vi "Write Sigle Dword.vi"(8 "error in (no error)":errorcluster, 10 "Data":u32, 11 "Tags":string) -> (0 "error out":errorcluster, 2 "Boolean":bool, 3 "Siemens Ctr out":T1)   [LabVIEW 2014]
uses:
  Simatic S7.lvlib
panel:
  in  "file path (dialog if empty)":path caption="文件路径 （空时为对话框）"
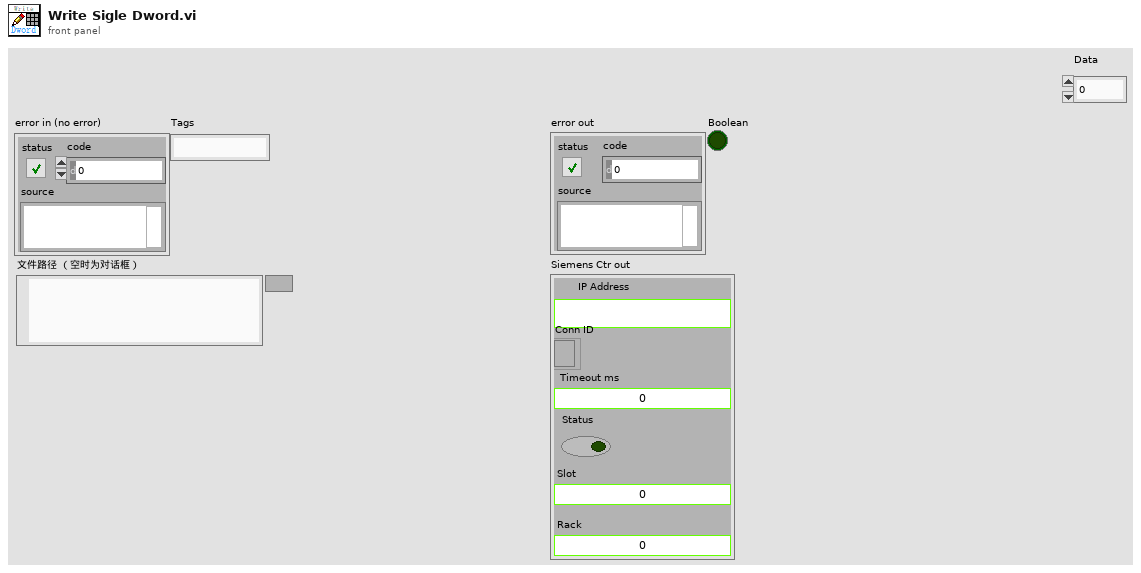
[diagram p1: front panel]
types:
  T1 = typedef "Simatic S7.lvlib/Siemens Ref.ctl" = cluster{"IP Address ":string, "Conn ID":refnum<k5>, "Timeout ms":i32, "Status":bool, "Slot":u16, "Rack":u16}
  T2 = typedef "Simatic S7.lvlib/Operation Siemens Ref.ctl" = enum16{"Init", "Add Ref", "Get Ref", "Set Error", "Close Close"}
  T3 = typedef "PLC Address.ctl" = cluster{"Address Areas":u8, "Data Type":enum8{"Bit", "Byte", "int", "Word", "Dint", "Dword", "Real", "String"}, "DB.No":u16, "Byte":u32, "Length":u16, "Item":u16}
  T4 = typedef "Semaphore RefNum" = refnum<k1>
  T5 = typedef "Simatic S7.lvlib/Op ip address.ctl" = enum16{"Init", "Add IP", "Get IP"}
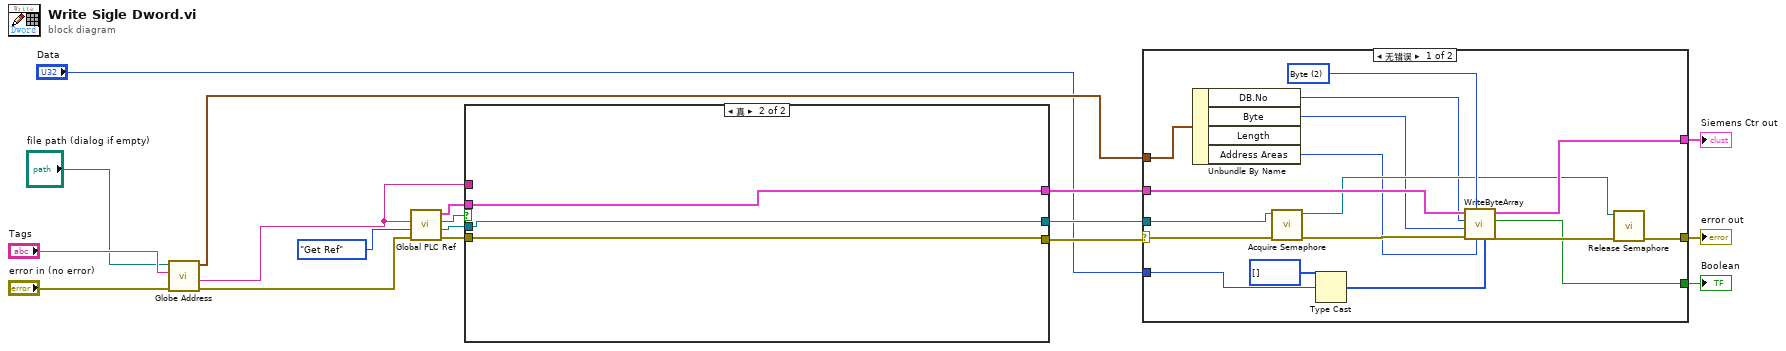
[diagram p0: block diagram]
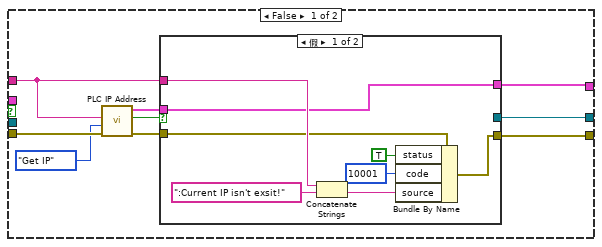
[diagram p3: hidden frame]
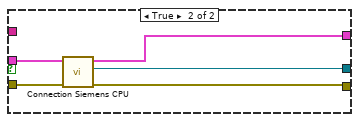
[diagram p4: hidden frame]
diagram:
  n1 = call "Globe Address.vi"("error in (no error)"="error in (no error)", "Tag"="Tags", "file path (dialog if empty)"="file path (dialog if empty)") -> ("error out"=w9:errorcluster, "IP"=w8:string, "ddress"=w6:T3)  [unwired: 5 in, 1 out]
  n2 = call "Global PLC Ref.vi"("error in (no error)"=w9, "Operation Siemens Ref"=Operation_Siemens_Ref."Get Ref", "IP Address"=w8) -> ("error out"=w16:errorcluster, "semaphore"=w14:T4, "Boolean"=w17:bool, "Siemens Ctr out"=w15:T1)  [unwired: 4 in, 1 out]
  n3 = case shown="真" w17 {
    tunnel: w16 -> [w27 w43]
    tunnel: w8 -> [w23 _]
    tunnel: [w21 w43] -> w13
    tunnel: [w20 w41] -> w12
    tunnel: [w19 w42] -> w11
    tunnel: w15 -> [_ w42]
    tunnel: w14 -> [_ w41]
    frame False {
      n4 = call "PLC IP Address.vi"("error in (no error)"=w27, "Operationip"=Op_ip_address."Get IP", "IP Address"=w23) -> ("error out"=w24:errorcluster, "Boolean"=w25:bool, "Siemens Ctr out"=w22:T1)  [unwired: 6 in]
      n5 = case shown="假" w25 {
        tunnel: w24 -> [w33 w40]
        tunnel: w23 -> [w34 _]
        tunnel: w22 -> [w28 w39]
        tunnel: [w29 w38] -> w21
        tunnel: [_ w37] -> w20
        tunnel: [w28 w36] -> w19
        frame False {
          n6 = Concatenate Strings(w34, ":Current IP isn't exsit!") -> (w31:string)
          n7 = Bundle By Name(cluster=w33, "status"=TRUE, "code"=10001, "source"=w31) -> (w29:errorcluster)
        }
        frame True {
          n8 = call "Connection Siemens CPU.vi"("error in (no error)"=w40, "Siemens Ctr in"=w39) -> ("error out"=w38:errorcluster, "semaphore"=w37:T4, "Siemens Ctr out"=w36:T1)  [unwired: 7 in]
        }
      }
    }
    frame True {
    }
  }
  n9 = case shown="无错误" w13 {
    selector: w13 -> [w60 w62]
    tunnel: w12 -> [w55 _]
    tunnel: w11 -> [w58 w61]
    tunnel: w6 -> [w57 _]
    tunnel: [w52 w62] -> w5
    tunnel: [w54 w61] -> w4
    tunnel: [w50 _] -> w2
    tunnel: "Data" -> [w45 _]
    frame No Error {
      w56 = u8 2 items=["Boolen"=1, "Byte"=2] ("Bit/Byte")
      n10 = Unbundle By Name(w57) -> ("DB.No"=w48:u16, "Byte"=w47:u32, "Address Areas"=w49:u8)  [unwired: 1 out]
      n11 = call <vilib>:"Acquire Semaphore.vi"("error in (no error)"=w60, "semaphore"=w55) -> ("error out"=w59:errorcluster, "semaphore out"=w51:T4)  [unwired: 3 in, 1 out]
      n12 = Type Cast(type=u8[] [], x=w45) -> (*(type *) &x=w44:u8[])
      n13 = call "WriteByteArray.vi"("Input"=w44, "Address Areas"=w49, "Bit/Byte"=w56, "error in (no error)"=w59, "Offset"=w47, "#DB No."=w48, "Siemens Ctr in"=w58) -> ("error out (no error)"=w53:errorcluster, "Data valid?"=w50:bool, "Siemens Ctr out"=w54:T1)  [unwired: 1 in, 1 out]
      n14 = call <vilib>:"Release Semaphore.vi"("error in (no error)"=w53, "semaphore"=w51) -> ("error out"=w52:errorcluster)  [unwired: 4 in, 1 out]
    }
    frame Error {
    }
  }
  "error out" <- w5
  "Siemens Ctr out" <- w4
  "Boolean" <- w2
